vi "main.vi"() -> ()   [LabVIEW 2025, in "Simple MCP Server.lvlib"]
doc: "This is a simple MCP server demo. Server is started, a tool is added and then the applications stays active and listens for an MCP client to connect and execute the \"Get System Stats.vi\".\n\nTo use the MCP Server, add this code to your claude_desktop_config.json (or other mcp config file for other clients):"
uses:
  Simple MCP Server.lvlib
  <vilib>/jgoebel/LabVIEW MCP Server SDK/MCP Server.lvlib
panel:
  out "String":string
  in  "stop":bool
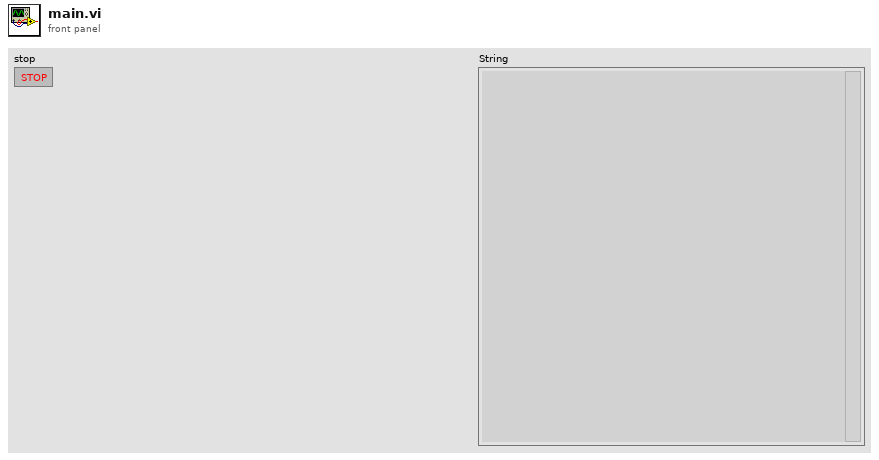
[diagram p1: front panel]
types:
  T1 = typedef "MCP Server.lvlib/User Events.ctl" = cluster{"onError":refnum<user-event>, "onLog":refnum<user-event>, "onConnect":refnum<user-event>, "onToolsList":refnum<user-event>, "onToolsCall":refnum<user-event>, "onNotification":refnum<user-event>, "onTool":refnum<user-event>, "onRpc":refnum<user-event>}
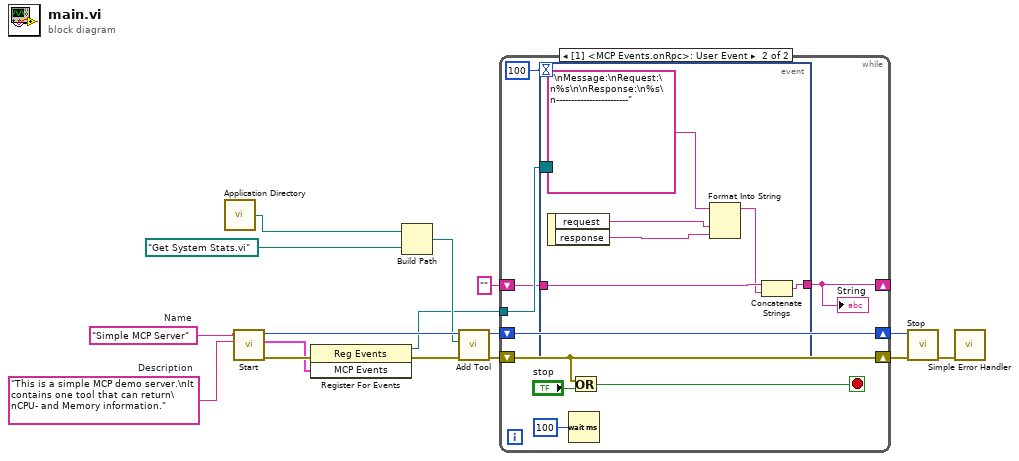
[diagram p0: block diagram]
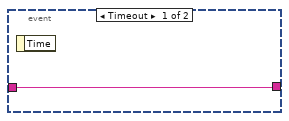
[diagram p2: hidden frame]
diagram:
  w9 = "This is a simple MCP demo server.\nIt contains one tool that can return\nCPU- and Memory information."  # Description
  w10 = "Simple MCP Server"  # Name
  n1 = call <vilib>:"Application Directory.vi"() -> ("Application Directory"=w8:path)
  n2 = call <vilib>:"Start.vi"("Description"=w9, "Name"=w10) -> ("error out"=w16:errorcluster, "MCP Events"=w2:T1, "id out"=w15:i32)  [unwired: 7 in]
  n3 = register-events(error in=w16, w2) -> (reference out=w3:refnum<event-registration>, error out=w4:errorcluster)  [unwired: 1 in]
  n4 = Build Path(base path=w8, name or relative path=path "Get System Stats.vi") -> (appended path=w6:path)
  n5 = call <vilib>:"Add Tool.vi"("error in (no error)"=w4, "vi path"=w6, "id"=w15) -> ("error out"=w14:errorcluster, "id out"=w12:i32)  [unwired: 7 in]
  n6 = while {
    shift-right: [w22] -> w13
    shift-left: w14 -> [w22]
    shift-right: [w25] -> w11
    shift-left: w12 -> [w25]
    tunnel: w3 -> [w20]
    shift-right: [w18] -> _
    shift-left: "" -> [w19]
    stop <- w23 stop-if-true
    n7 = event shown="[1] <MCP Events.onRpc>: User Event" {
      selector: w20 -> [_ _]
      dyn-events: _ -> [_ _]
      timeout: 100 -> [_ _]
      tunnel: [w26 w28] -> w18
      tunnel: w19 -> [w26 w29]
      event Timeout {
        n8 = event-data() -> ()  [unwired: 1 in, 1 out]
      }
      event User Event {
        n9 = event-data() -> ("request"=w32:string, "response"=w31:string)  [unwired: 1 in]
        n10 = Format Into String(format string="\nMessage:\nRequest:\n%s\n\nResponse:\n%s\n------------------------", w32, w31) -> (resulting string=w27:string)  [unwired: 2 in, 1 out]
        n11 = Concatenate Strings(w29, w27) -> (w28:string)
      }
    }
    "String" <- w18
    n12 = Wait (ms)(milliseconds to wait=u32 100) -> ()  [unwired: 1 out]
    n13 = Or(x=w22, y="stop") -> (x .or. y?=w23:bool)
  }
  n14 = call <vilib>:"Stop.vi"("error in (no error)"=w13, "id"=w11) -> ("error out"=w5:errorcluster)  [unwired: 9 in]
  n15 = call <vilib>:"Simple Error Handler.vi"("error in (no error)"=w5) -> ()  [unwired: 4 in, 5 out]
